vi "cpIMG.vi"(6 "线程":i32=4, 8 "error in (no error)":errorcluster caption="错误输入（无错误）", 11 "EPUB 输入":refnum<class "EPUB.lvclass">) -> (0 "error out":errorcluster caption="错误输出", 3 "EPUB 输出":refnum<class "EPUB.lvclass">)   [LabVIEW 2016, in "EPUB.lvclass"]
uses:
  EPUB.lvclass
  EPUB.lvclass/EPUB.ctl
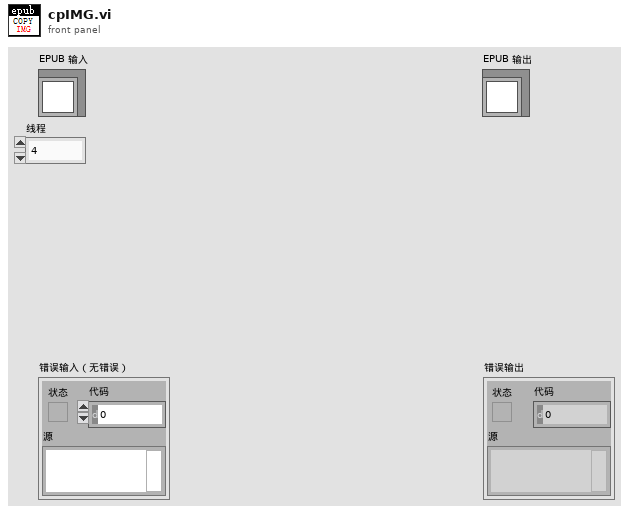
[diagram p1: front panel]
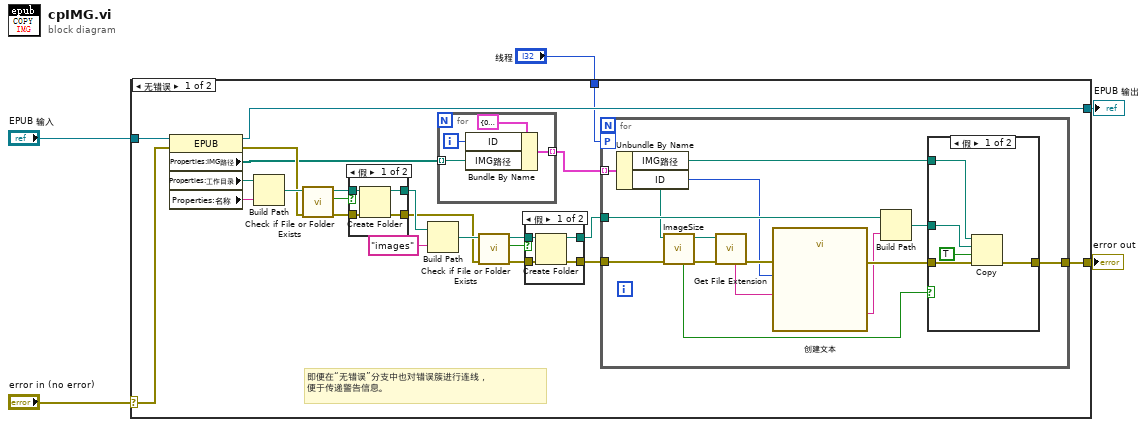
[diagram p0: block diagram]
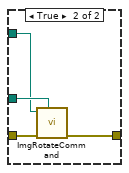
[diagram p2: hidden frame]
diagram:
  n1 = case shown="无错误" "error in (no error)" {
    selector: "error in (no error)" -> [w26 w68]
    tunnel: [w27 w69] -> w3
    tunnel: "EPUB 输入" -> [w28 w69]
    tunnel: [w9 w68] -> w2
    tunnel: "线程" -> [w6 _]
    frame No Error {
      # "即便在“无错误”分支中也对错误簇进行连线，\n便于传递警告信息。"
      n2 = property class="EPUB"(reference=w28, error in=w26) -> (reference out=w27:refnum<class "EPUB.lvclass">, error out=w22:errorcluster, "Properties:IMG路径"=w8:path[], "Properties:工作目录"=w24:path, "Properties:名称"=w25:string)
      n3 = Build Path(base path=w24, name or relative path=w25) -> (appended path=w23:path)
      n4 = call <vilib>:"Check if File or Folder Exists.vi"("error in (no error)"=w22, "path"=w23) -> ("error out"=w21:errorcluster, "file or folder exists?"=w19:bool, "dup path"=w20:path)  [unwired: 7 in]
      n5 = case shown="假" w19 {
        tunnel: w21 -> [w65 w66]
        tunnel: w20 -> [w64 w67]
        tunnel: [w63 w67] -> w18
        tunnel: [w62 w66] -> w15
        frame False {
          n6 = Create Folder(path (use dialog)=w64, error in=w65) -> (created path=w63:path, error out=w62:errorcluster)  [unwired: 1 in, 1 out]
        }
        frame True {
        }
      }
      n7 = Build Path(base path=w18, name or relative path="images" ("名称或相对路径")) -> (appended path=w16:path)
      n8 = for {
        tunnel: w8 -> [w31] mode=indexing
        tunnel: [w29] -> w7 mode=indexing
        i -> [w32]
        n9 = Bundle By Name(cluster=cluster{"ID":i32, "IMG路径":path} {"ID"=0, "IMG路径"=path ""} ("输出簇"), "ID"=w32, "IMG路径"=w31) -> (w29:cluster{"ID":i32, "IMG路径":path})
      }
      n10 = call <vilib>:"Check if File or Folder Exists.vi"("error in (no error)"=w15, "path"=w16) -> ("error out"=w14:errorcluster, "file or folder exists?"=w12:bool, "dup path"=w13:path)  [unwired: 7 in]
      n11 = case shown="假" w12 {
        tunnel: w14 -> [w59 w60]
        tunnel: w13 -> [w58 w61]
        tunnel: [w57 w61] -> w11
        tunnel: [w56 w60] -> w10
        frame False {
          n12 = Create Folder(path (use dialog)=w58, error in=w59) -> (created path=w57:path, error out=w56:errorcluster)  [unwired: 1 in, 1 out]
        }
        frame True {
        }
      }
      n13 = for {
        tunnel: w11 -> [w39]
        tunnel: w10 -> [w45]
        tunnel: w7 -> [w36] mode=indexing
        tunnel: [w46] -> w9
        workers-P: w6 -> [_]
        n14 = Unbundle By Name(w36) -> ("IMG路径"=w34:path, "ID"=w33:i32)
        n15 = call "ImageSize.vi"("Error in"=w45, "filename"=w34) -> ("Error out"=w38:errorcluster, "filename out"=w37:path, "landscape"=w35:bool)  [unwired: 5 in, 2 out]
        n16 = call <vilib>:"Get File Extension.vi"("error in (no error)"=w38, "file"=w37) -> ("error out"=w43:errorcluster, "unmodified file extension"=w42:string)  [unwired: 5 in, 3 out]
        n17 = call "创建文本"("idx"=w33, "img_ext"=w42, "error in (no error)"=w43) -> ("Result"=w40:string, "error out"=w44:errorcluster)  [unwired: 11 in]
        n18 = Build Path(base path=w39, name or relative path=w40) -> (appended path=w41:path)
        n19 = case shown="假" w35 {
          tunnel: [w51 w54] -> w46
          tunnel: w44 -> [w49 w55]
          tunnel: w41 -> [w48 w53]
          tunnel: w34 -> [w47 w52]
          frame False {
            n20 = Copy(8:w49, 9:TRUE ("覆盖(F)"), 10:w48, 11:w47) -> (0:w51:errorcluster)  [unwired: 1 in, 2 out]
          }
          frame True {
            n21 = call "ImgRotateCommand.vi"("OutputFiles"=w53, "Error in"=w55, "ImgPath"=w52) -> ("Error out"=w54:errorcluster)  [unwired: 6 in, 2 out]
          }
        }
      }
    }
    frame Error {
    }
  }
  "error out" <- w2
  "EPUB 输出" <- w3
